vi "PI_Regulering.vi"(8 "k_i":dbl, 9 "k_p":dbl, 10 "SP":dbl, 11 "DATA":dbl) -> (0 "p_pi":dbl, 1 "i_pi":dbl, 2 "e(t)":dbl, 3 "u_pi":dbl)   [LabVIEW 2022 SP3]
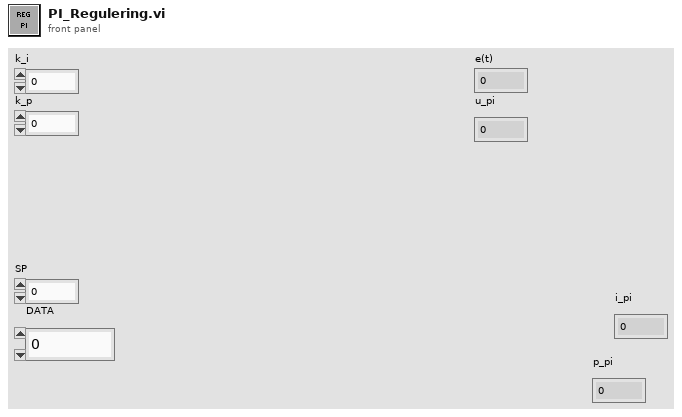
[diagram p1: front panel]
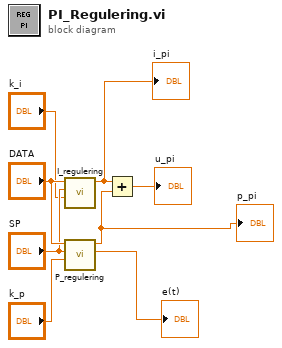
[diagram p0: block diagram]
diagram:
  n1 = call "I_regulering.vi"("k_i"="k_i", "SP"="SP", "DATA"="DATA") -> ("u_i"=w2:dbl)  [unwired: 6 in, 2 out]
  "i_pi" <- w2
  n2 = call "P_regulering.vi"("k_p"="k_p", "SP"="SP", "DATA"="DATA") -> ("e(t)"=→"e(t)":dbl, "u_p"=w1:dbl)  [unwired: 6 in, 1 out]
  "p_pi" <- w1
  n3 = Add(x=w2, y=w1) -> (x+y=→"u_pi":dbl)
